vi "Check for Viewer Requests.vi"(8 "error in (no error)":errorcluster, 11 "Data Server Thread in":refnum<class "Data Server Thread.lvclass">) -> (0 "error out":errorcluster, 3 "Data Server Thread out":refnum<class "Data Server Thread.lvclass">)   [LabVIEW 2017, in "DSF Core.lvlib" / "Data Server Thread.lvclass"]
uses:
  Data Server Thread.lvclass
  Data Server Thread.lvclass/Data Server Thread.ctl
  Typedefs/DSF Buffer Type.ctl
  <vilib>/NI/Memory Manager/Classes/Pointer/Pointer.lvclass/Pointer.ctl
  <vilib>/NI/Memory Manager/Classes/Pointer/Get Address.vi
  <vilib>/NI/Memory Manager/Classes/Pointer/Encapsulate.vi
  <vilib>/NI/Memory Manager/Classes/Pointer/Check Null Pointer.vi
  <vilib>/NI/Memory Manager/Classes/Pointer/Check Length.vi
  <vilib>/NI/Memory Manager/Classes/Pointer/Set Size.vi
  <vilib>/NI/Memory Manager/Classes/Pointer/Set Address.vi
  <vilib>/NI/Memory Manager/Classes/Pointer/Set Internal.vi
  <vilib>/NI/Memory Manager/Classes/Pointer/Errors.vi
  <vilib>/NI/Memory Manager/Classes/Pointer/Null Pointer.vi
  <vilib>/NI/Memory Manager/Classes/Pointer/Is Null.vi
  <vilib>/NI/Memory Manager/Classes/Pointer/Get Size.vi
  <vilib>/NI/Memory Manager/Classes/Pointer/Check Bounds (Pointer).vi
  <vilib>/NI/Memory Manager/Classes/Pointer/Create Error.vi
  <vilib>/NI/Memory Manager/Classes/Pointer/Out of Bounds.vi
  <vilib>/NI/Memory Manager/Constants/Constants.vi
  <vilib>/NI/Memory Manager/Constants/Library Name.vi
  <vilib>/NI/Memory Manager/Classes/Pointer/Pointer Error Info.vi
  <vilib>/NI/Memory Manager/Constants/Pointer Class Name.vi
  <vilib>/NI/Memory Manager/Classes/Pointer/Write Pointer Size to Error.vi
  Buffer/Buffer.lvclass
  C:/Program Files (x86)/National Instruments/LabVIEW 2017/vi.lib/NI/Memory Manager/Classes/Pointer/Pointer.lvclass
  <vilib>/NI/Memory Manager/VIs/New Error Cluster.vi
  <vilib>/NI/Memory Manager/VIs/New Error Cluster (512B).vi
  <vilib>/NI/Memory Manager/VIs/Set Error Status.vi
  <vilib>/NI/Memory Manager/VIs/Set Error Code.vi
  <vilib>/NI/Memory Manager/VIs/Set Error Source.vi
  <vilib>/NI/Memory Manager/VIs/Write String to Source.vi
  <vilib>/NI/Memory Manager/VIs/Write Numeric to Source.vi
  <vilib>/NI/Memory Manager/VIs/Write Numeric Scalar to Source (Base10 U64).vi
  Buffer Map/Buffers Map.lvclass
  DSF Core.lvlib
  <vilib>/NI/Memory Manager/Classes/Pointer/Pointer.lvclass
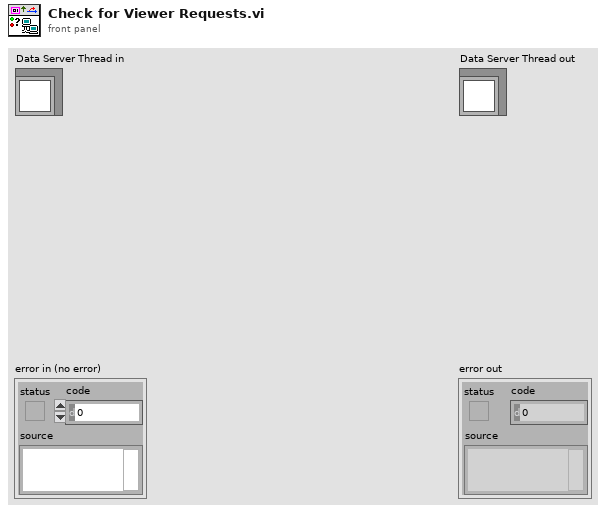
[diagram p1: front panel]
types:
  T1 = typedef "DSF Core.lvlib/DSF Buffer Type.ctl" = enum16{"Engine", "String"}
  T2 = typedef "DSF Core.lvlib/Data Server Thread.lvclass/Viewer Data.ctl" = cluster{"remote address":string, "remote port":u16, "connection ID":refnum<k5>, "Buffer":refnum<class "Buffer.lvclass">}
  T3 = typedef "DSF Core.lvlib/Data Server Thread.lvclass/Buffer Descriptor.ctl" = cluster{"buffer type":T1, "plugin id":i32, "group id":i32, "transfer id":i32, "offset (0)":u64, "length (-1: rest)":i64}
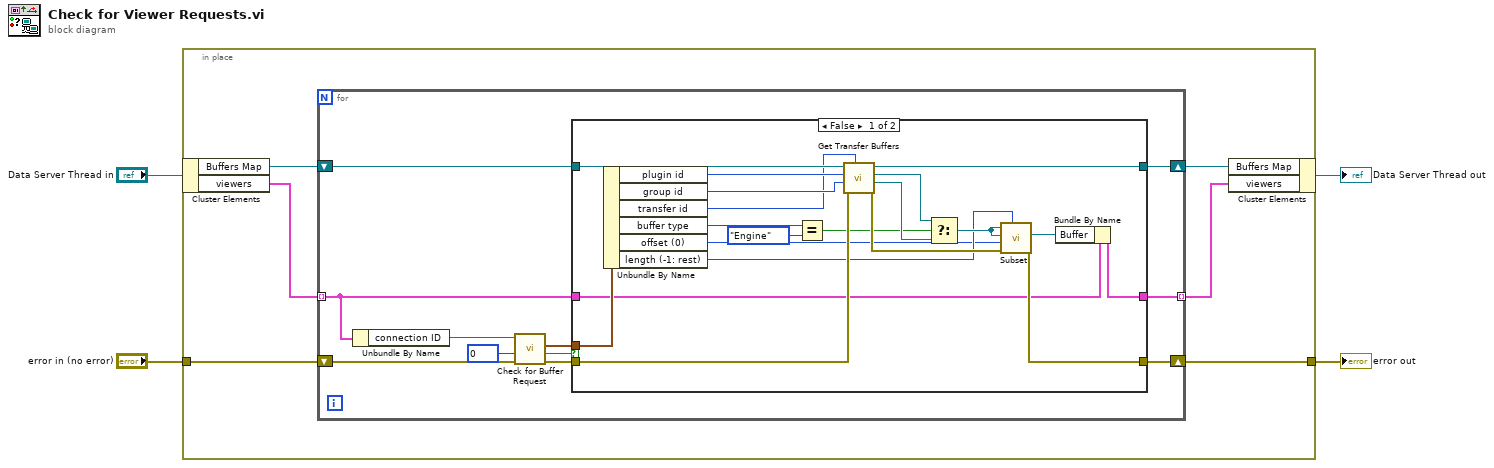
[diagram p0: block diagram]
diagram:
  n1 = in-place {
    in-place-border: [w10] -> w4
    in-place-border: "error in (no error)" -> [w9]
    n2 = in-place-cluster #1("Data Server Thread in") -> ("Buffers Map"=w7:refnum<class "Buffers Map.lvclass">, "viewers"=w8:T2[])
    n3 = for {
      tunnel: w8 -> [w18] mode=indexing
      shift-right: [w12] -> w10
      shift-left: w9 -> [w21]
      tunnel: [w15] -> w5 mode=indexing
      shift-right: [w14] -> w6
      shift-left: w7 -> [w16]
      n4 = Unbundle By Name(w18) -> ("connection ID"=w20:refnum<k5>)
      n5 = call "Check for Buffer Request.vi"("error in (no error)"=w21, "timeout ms (25000)"=0, "connection ID in"=w20) -> ("error out"=w13:errorcluster, "timed out?"=w17:bool, "buffer descriptor"=w11:T3)  [unwired: 5 in, 1 out]
      n6 = case shown="False" w17 {
        tunnel: w18 -> [w25 w43]
        tunnel: w11 -> [w39 _]
        tunnel: w16 -> [w40 w42]
        tunnel: [w24 w43] -> w15
        tunnel: [w38 w42] -> w14
        tunnel: w13 -> [w35 w44]
        tunnel: [w26 w44] -> w12
        frame False {
          n7 = Unbundle By Name(w39) -> ("plugin id"=w37:i32, "group id"=w36:i32, "transfer id"=w22:i32, "buffer type"=w27:T1, "offset (0)"=w28:u64, "length (-1: rest)"=w29:i64)
          n8 = Equal?(x=w27, y=DSF_Buffer_Type."Engine") -> (x = y?=w31:bool)
          n9 = call "Get Transfer Buffers.vi"("transfer id"=w22, "error in (no error)"=w35, "group id"=w36, "plugin id"=w37, "Buffers Map in"=w40) -> ("error out"=w41:errorcluster, "string Buffer"=w33:refnum<class "Buffer.lvclass">, "engine Buffer"=w32:refnum<class "Buffer.lvclass">, "Buffers Map out"=w38:refnum<class "Buffers Map.lvclass">)  [unwired: 3 in]
          n10 = Select(t=w32, s=w31, f=w33) -> (s? t:f=w30:refnum<class "Buffer.lvclass">)
          n11 = call <vilib>:"Subset.vi"("length (-1: rest)"=w29, "error in (no error)"=w41, "offset (0)"=w28, "subset Pointer type"=w30, "base Pointer in"=w30) -> ("error out"=w26:errorcluster, "subset Pointer"=w23:refnum<class "Buffer.lvclass">)  [unwired: 3 in, 2 out]
          n12 = Bundle By Name(cluster=w25, "Buffer"=w23) -> (w24:T2)
        }
        frame True {
        }
      }
    }
    n13 = in-place-cluster #1("Buffers Map"=w6, "viewers"=w5) -> (→"Data Server Thread out":refnum<class "Data Server Thread.lvclass">)
  }
  "error out" <- w4
